vi "DAQNavi Read (Digital 1D Wfm NChan NSamp).vi"(8 "error in (no error)":errorcluster, 9 "number of samples per channel to read":u32=1000, 10 "timeout":dbl=10.0 format="%0.2f", 11 "task in":i32) -> (0 "error out":errorcluster, 2 "data":digitalwaveform[](array[waveform]), 3 "task out":i32)   [LabVIEW 2020]
uses:
  DAQNavi_LV.dll
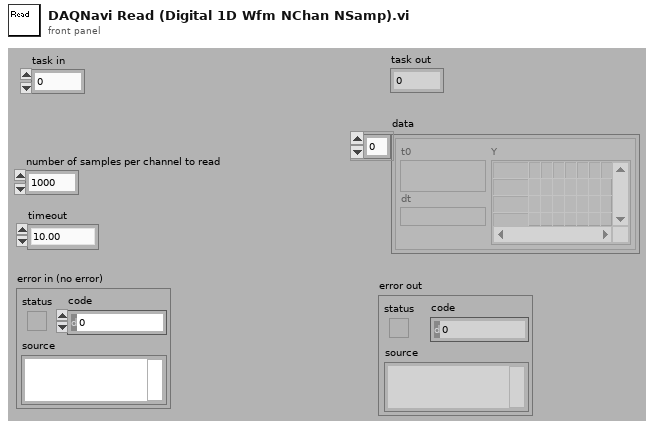
[diagram p1: front panel]
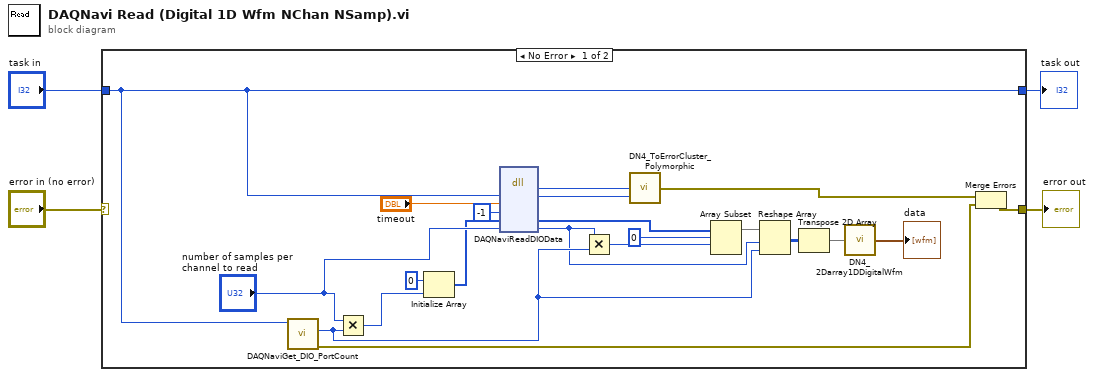
[diagram p0: block diagram]
diagram:
  n1 = case shown="No Error" "error in (no error)" {
    selector: "error in (no error)" -> [_ w26]
    tunnel: "task in" -> [w21 w27]
    tunnel: [w21 w27] -> w2
    tunnel: [w19 w26] -> w1
    frame No Error {
      n2 = call "DAQNaviGet_DIO_PortCount.vi"("task in"=w21) -> ("error out"=w17:errorcluster, "port count"=w13:i32)  [unwired: 1 in, 8 out]
      n3 = Multiply(x="number of samples per channel to read", y=w13) -> (x*y=w20:u32)
      n4 = Initialize Array(u8 0 ("element"), w20) -> (w10:u8[])
      n5 = dll-call lib="DAQNavi_LV.dll" fn="DAQNaviReadDIOData"("taskID"=w21, "timeout"="timeout", "portBit"=-1, "portData"=w10, "samples"="number of samples per channel to read") -> ("return type"=w23:i32, "taskID"=w6:i32, "portData"=w9:u8[], "samples"=w12:u32)  [unwired: 5 in, 2 out]
      n6 = Multiply(x=w12, y=w13) -> (x*y=w14:u32)
      n7 = call "DN4_ToErrorCluster_Polymorphic.vi"("task id"=w6, "error code"=w23) -> ("error out"=w18:errorcluster)  [unwired: 3 out]
      n8 = Array Subset(array=w9, index=0, length=w14) -> (w16:u8[])
      n9 = Reshape Array(w16, w12, w13) -> (w15:u8[][])
      n10 = Transpose 2D Array(2D array=w15) -> (transposed array=w8:u8[][])
      n11 = call "DN4_2Darray1DDigitalWfm.vi"("data"=w8) -> ("1D Wfm"=→"data":digitalwaveform[])
      n12 = Merge Errors(w18, w17) -> (w19:errorcluster)
    }
    frame Error {
    }
  }
  "task out" <- w2
  "error out" <- w1
